vi "Vision.vi"() -> ()   [LabVIEW 2011]
panel:
  in  "Boolean":bool
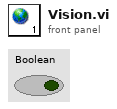
[diagram p1: front panel]
diagram:
